vi "NMRvmeCard5.vi"() -> ()   [LabVIEW 2013]
uses:
  <vilib>/Utility/file.llb/Read From Spreadsheet File (DBL).vi
  <vilib>/Analysis/NI_AALBase.lvlib
panel:
  out "Diff Sigma":dbl=0.0014967762883509395 format="%#_13g"
  out "Peak center (MHz)":sgl=213.00838 format="%.3f"
  out "Peak width (MHz)":sgl=0.03243152 format="%.5f"
  in  "Max":bool
  in  "Logoffset (V)":dbl=-5.996000000000003 min=-9.0 max=0.0 step=0.0005 format="%_5g"
  in  "Phase (V)":dbl=6.500000000000002 min=0.0 max=9.0 step=0.0005 format="%_5g"
  out "Telnet error out":errorcluster
  in  "Real/Quad Q curve":bool=TRUE
  out "Temperature (C)":dbl(graph)=27.0
  out "+3V supply":dbl=3.245 format="%_4g"
  out "Temp (C)":dbl=27.0 format="%_4g"
  in  "RemovePed":bool=TRUE
  in  "IF / LOG Det":bool
  in  "Q curve file":string="realback212a.txt"
  out "File name 2":string="C:\\users\\plm\\Desktop\\rssmt\\realback212a.txt"
  in  "AutoTune":bool
  out "RF OK":bool=TRUE
  out "Peak area (V-MHz)":sgl=0.00324335 format="%.5f"
  in  "Gauss Fit":bool
  out "NMR Graph + Fit":cluster{cluster{dbl, "Numeric":dbl}[]}[](graph)=[{[{212.6, "Numeric"=-0.005730750000000197}, {212.60999999999999, "Numeric"=-0.006890750000001482}, {212.62, "Numeric"=-0.003986749999998765}, {212.63, "Numeric"=-0.004218750000000024}, {212.64, "Numeric"=-0.003786750000001219}, {212.65, "Numeric"=-0.004290749999998711}, {212.66, "Numeric"=-0.005430749999999876}, {212.67, "Numeric"=-0.006406750000000973}, {212.68, "Numeric"=-0.005218749999998682}, {212.69, "Numeric"=-0.004966749999999748}, {212.7, "Numeric"=-0.003950750000000758}, {212.71, "Numeric"=-0.0042707499999986775}, {212.72, "Numeric"=-0.004126749999999656}, {212.73, "Numeric"=-0.004318750000000561}, {212.74, "Numeric"=-0.003946750000001408}, {212.75, "Numeric"=-0.00391074999999958}, {212.76, "Numeric"=-0.003910750000000397}, {212.77, "Numeric"=-0.002246750000001148}, {212.78, "Numeric"=-0.002018749999999532}, {212.79, "Numeric"=-0.0012267500000002545}, {212.8, "Numeric"=-0.0017707500000009122}, {212.81, "Numeric"=-0.0019507499999995084}, {212.82, "Numeric"=-0.002066750000000136}, {212.82999999999998, "Numeric"=-0.0013187500000007004}, {212.84, "Numeric"=0.00039325000000048956}, {212.85, "Numeric"=0.00016924999999995416}, {212.85999999999999, "Numeric"=0.0010092499999994845}, {212.87, "Numeric"=1.3250000000461677e-05}, {212.88, "Numeric"=0.0003812500000000196}, {212.89, "Numeric"=0.0014132499999996448}, {212.9, "Numeric"=0.002609250000000409}, {212.91, "Numeric"=0.0036692500000000622}, {212.92, "Numeric"=0.0037932499999997803}, {212.93, "Numeric"=0.0045812500000003325}, {212.94, "Numeric"=0.005733250000000078}, {212.95, "Numeric"=0.007449249999999889}, {212.96, "Numeric"=0.012029250000000227}, {212.97, "Numeric"=0.02267325000000007}, {212.98, "Numeric"=0.03378124999999998}, {212.99, "Numeric"=0.033853249999999946}, {213.0, "Numeric"=0.024589250000000035}, {213.01, "Numeric"=0.021789250000000034}, {213.02, "Numeric"=0.0198532500000001}, {213.03, "Numeric"=0.016981249999999976}, {213.04, "Numeric"=0.01617325000000007}, {213.05, "Numeric"=0.016929250000000225}, {213.06, "Numeric"=0.01484924999999989}, {213.07, "Numeric"=0.015133250000000077}, {213.08, "Numeric"=0.01338125000000033}, {213.09, "Numeric"=0.00949324999999978}, {213.1, "Numeric"=0.007269250000000061}, {213.11, "Numeric"=0.0051092500000004095}, {213.12, "Numeric"=0.004413249999999646}, {213.13, "Numeric"=0.004781250000000021}, {213.14000000000001, "Numeric"=0.0035132500000004613}, {213.15, "Numeric"=0.0027092499999994838}, {213.16, "Numeric"=0.003069249999999955}, {213.17000000000002, "Numeric"=0.004893250000000488}, {213.18, "Numeric"=0.0052812499999992995}, {213.19, "Numeric"=0.0037332499999998625}, {213.2, "Numeric"=0.002549250000000493}, {213.21, "Numeric"=0.003029249999999089}, {213.22, "Numeric"=0.0034732499999997465}, {213.23, "Numeric"=0.0036812500000004663}, {213.24, "Numeric"=0.0035532500000012594}, {213.25, "Numeric"=0.003889249999999604}, {213.26, "Numeric"=0.00258925000000042}, {213.27, "Numeric"=0.0017532500000013032}, {213.28, "Numeric"=0.0021812499999994397}, {213.29, "Numeric"=0.002873250000000347}, {213.3, "Numeric"=0.0024292500000013236}, {213.31, "Numeric"=0.0036492499999992442}, {213.32, "Numeric"=0.003733250000000251}, {213.33, "Numeric"=0.003981250000001318}, {213.34, "Numeric"=0.004593249999999026}, {213.35, "Numeric"=0.0042692500000001245}, {213.36, "Numeric"=0.004509250000001291}, {213.37, "Numeric"=0.004313249999998781}, {213.38, "Numeric"=0.005381249999999974}, {213.39000000000001, "Numeric"=0.006313250000001235}, {213.4, "Numeric"=0.005309249999998517}]}]
  in  "Amp of Q curve":dbl=1.8000000000000034 min=0.0 max=29.0 step=0.01 format="%_3f"
  in  "Subtract Q curve":bool=TRUE
  out "Pedestal Offset":dbl(graph)=0.005806249999999974
  out "Pedestal Difference":dbl(graph)=0.007663500000000241
  out "# Good Spectra":i32=50
  in  "Quality cuts":bool=TRUE
  out "Pedestal OK":bool=TRUE
  out "Sweep #":i32=22
  out "1st Sweep":bool
  out "ADC volts OK":bool=TRUE
  out "Peak Height Distribution":cluster{"Y":dbl[], "Y":dbl[]}[](graph)=[{"Y"=[0.02977452083333331, 0.029831895833333313, 0.02988927083333331, 0.029946645833333313, 0.03000402083333331, 0.030061395833333313, 0.03011877083333331, 0.03017614583333331, 0.030233520833333312, 0.03029089583333331, 0.030348270833333312, 0.03040564583333331, 0.030463020833333312, 0.03052039583333331, 0.030577770833333313, 0.03063514583333331, 0.030692520833333313, 0.03074989583333331, 0.030807270833333313, 0.03086464583333331, 0.03092202083333331, 0.030979395833333312, 0.03103677083333331, 0.031094145833333312, 0.03115152083333331, 0.031208895833333312, 0.03126627083333331, 0.03132364583333331, 0.031381020833333315, 0.03143839583333331, 0.03149577083333331, 0.03155314583333331, 0.03161052083333331, 0.031667895833333314, 0.03172527083333331, 0.03178264583333331, 0.03184002083333331, 0.031897395833333314, 0.03195477083333331, 0.03201214583333331, 0.03206952083333331, 0.032126895833333315, 0.03218427083333331, 0.03224164583333331, 0.03229902083333331, 0.03235639583333331, 0.032413770833333314, 0.03247114583333331, 0.03252852083333331, 0.03258589583333331, 0.032643270833333314, 0.03270064583333331, 0.03275802083333331, 0.03281539583333331, 0.032872770833333315, 0.03293014583333331, 0.03298752083333331, 0.03304489583333331, 0.03310227083333331, 0.033159645833333314, 0.03321702083333331, 0.03327439583333331, 0.03333177083333331, 0.033389145833333314, 0.03344652083333331, 0.03350389583333331, 0.03356127083333331, 0.033618645833333315, 0.03367602083333331, 0.03373339583333331, 0.03379077083333331, 0.03384814583333331, 0.033905520833333314, 0.03396289583333331, 0.03402027083333331, 0.03407764583333331, 0.034135020833333314, 0.03419239583333331, 0.03424977083333331, 0.03430714583333331, 0.034364520833333315, 0.03442189583333331, 0.03447927083333331, 0.03453664583333331, 0.03459402083333331, 0.034651395833333314, 0.03470877083333331, 0.03476614583333331, 0.03482352083333331, 0.034880895833333314, 0.03493827083333331, 0.03499564583333331, 0.03505302083333331, 0.035110395833333315, 0.03516777083333331, 0.03522514583333331, 0.03528252083333331, 0.03533989583333331, 0.035397270833333314, 0.03545464583333331], "Y"=[1.0, 0.0, 0.0, 0.0, 1.0, 0.0, 1.0, 0.0, 0.0, 0.0, 0.0, 0.0, 0.0, 1.0, 0.0, 0.0, 0.0, 0.0, 0.0, 1.0, 0.0, 1.0, 0.0, 0.0, 0.0, 1.0, 1.0, 1.0, 0.0, 1.0, 0.0, 0.0, 0.0, 1.0, 1.0, 0.0, 1.0, 0.0, 2.0, 2.0, 4.0, 0.0, 2.0, 1.0, 1.0, 3.0, 0.0, 0.0, 1.0, 0.0, 1.0, 0.0, 1.0, 1.0, 1.0, 0.0, 0.0, 1.0, 1.0, 0.0, 1.0, 0.0, 1.0, 1.0, 0.0, 1.0, 1.0, 1.0, 0.0, 0.0, 0.0, 0.0, 0.0, 1.0, 2.0, 0.0, 0.0, 1.0, 1.0, 0.0, 0.0, 1.0, 1.0, 0.0, 0.0, 1.0, 0.0, 0.0, 0.0, 0.0, 0.0, 0.0, 0.0, 0.0, 0.0, 0.0, 0.0, 0.0, 0.0, 1.0]}]
  in  "# of Sweeps":i32=50
  out "S/N":dbl=25.80021937658381 format="%_3g"
  out "Peak mean (V)":dbl=0.03249358666666663 format="%_4g"
  out "Peak Height":dbl(graph)=0.033853249999999946
  in  "Raw Data":bool=TRUE
  in  "Tank RF":bool=TRUE
  in  "IF Atten (dB)":i8=3 min=0 max=31 step=1
  in  "IFoffset (V)":dbl=5.450461000000012 min=-0.0 max=9.0 step=0.001 format="%.4f"
  in  "Tune  (V)":dbl=0.3670000000000009 min=-0.5 max=8.0 step=0.001 format="%.4f"
  in  "Hi / Lo Gain":bool
  out "Voltage Array":sgl[](array[numeric])=[0.0296, 0.027, 0.0285, 0.0269, 0.026, 0.0242, 0.0218, 0.0196, 0.0196, 0.0187, 0.0186, 0.0172, 0.0163, 0.0151, 0.0145, 0.0136, 0.0127, 0.0135, 0.0129, 0.0129, 0.0116, 0.0107, 0.0099, 0.01, 0.0111, 0.0103, 0.0106, 0.0091, 0.009, 0.0096, 0.0104, 0.0111, 0.0109, 0.0114, 0.0123, 0.0138, 0.0182, 0.0287, 0.0397, 0.0397, 0.0304, 0.0276, 0.0257, 0.0229, 0.0222, 0.0231, 0.0212, 0.0217, 0.0202, 0.0166, 0.0147, 0.0129, 0.0126, 0.0134, 0.0126, 0.0123, 0.0132, 0.0156, 0.0166, 0.0157, 0.0152, 0.0164, 0.0176, 0.0186, 0.0193, 0.0205, 0.0201, 0.0202, 0.0216, 0.0233, 0.0239, 0.0262, 0.0274, 0.0288, 0.0306, 0.0315, 0.033, 0.0341, 0.0365, 0.0388, 0.0392] format="%.4f"
  in  "Invert Polarity":bool=TRUE
  out "Pedestal Diff (V)":sgl=0.0076635 format="%.3f"
  out "Peak amp (V)":sgl=0.03385325 format="%.3f"
  in  "Save Data to File":bool
  in  "RF Level (dBm)":dbl min=-10.0 max=10.0 step=0.1 format="%.2f"
  out "SMT error out":errorcluster
  out "Sample RMS (V)":dbl=0.0009444444444444443 format="%.4f"
  in  "# Sample/step":i32=80 min=1 max=5000 step=100
  in  "Step Width (MHz)":dbl=0.01 min=0.0 max=1000.0 step=0.0001 format="%.4f"
  in  "Freq Span (MHz)":dbl=0.8 min=0.0 max=3000.0 step=0.1 format="%.3f"
  in  "Center Freq (MHz)":dbl=213.0 min=0.005 max=6000.0 step=0.1 format="%.3f"
  in  "Sweep Mode":u16(ring)=3 items=["Off", "Single", "Auto", "Step"]
  in  "GPIB Addr (28)":refnum<visa-resource-name>="GPIB0::28::INSTR"
  # "E1039 Prototype NMR Control Panel"
  # "Settings"
  # "D\nA\nC"
  # "R\nF\n\nG\nE\nN \n\n+\n\nI\nF"
  # "A\nD\nC"
  # "I\n/\nO"
  # "D\nA\nT\nA\n\nA \nN\nA\nL\nY\nS\nI\nS"
  # "Results"
  # "A\nv\ne\nr\na\ng\ne"
  # "S\nw\ne\ne\np"
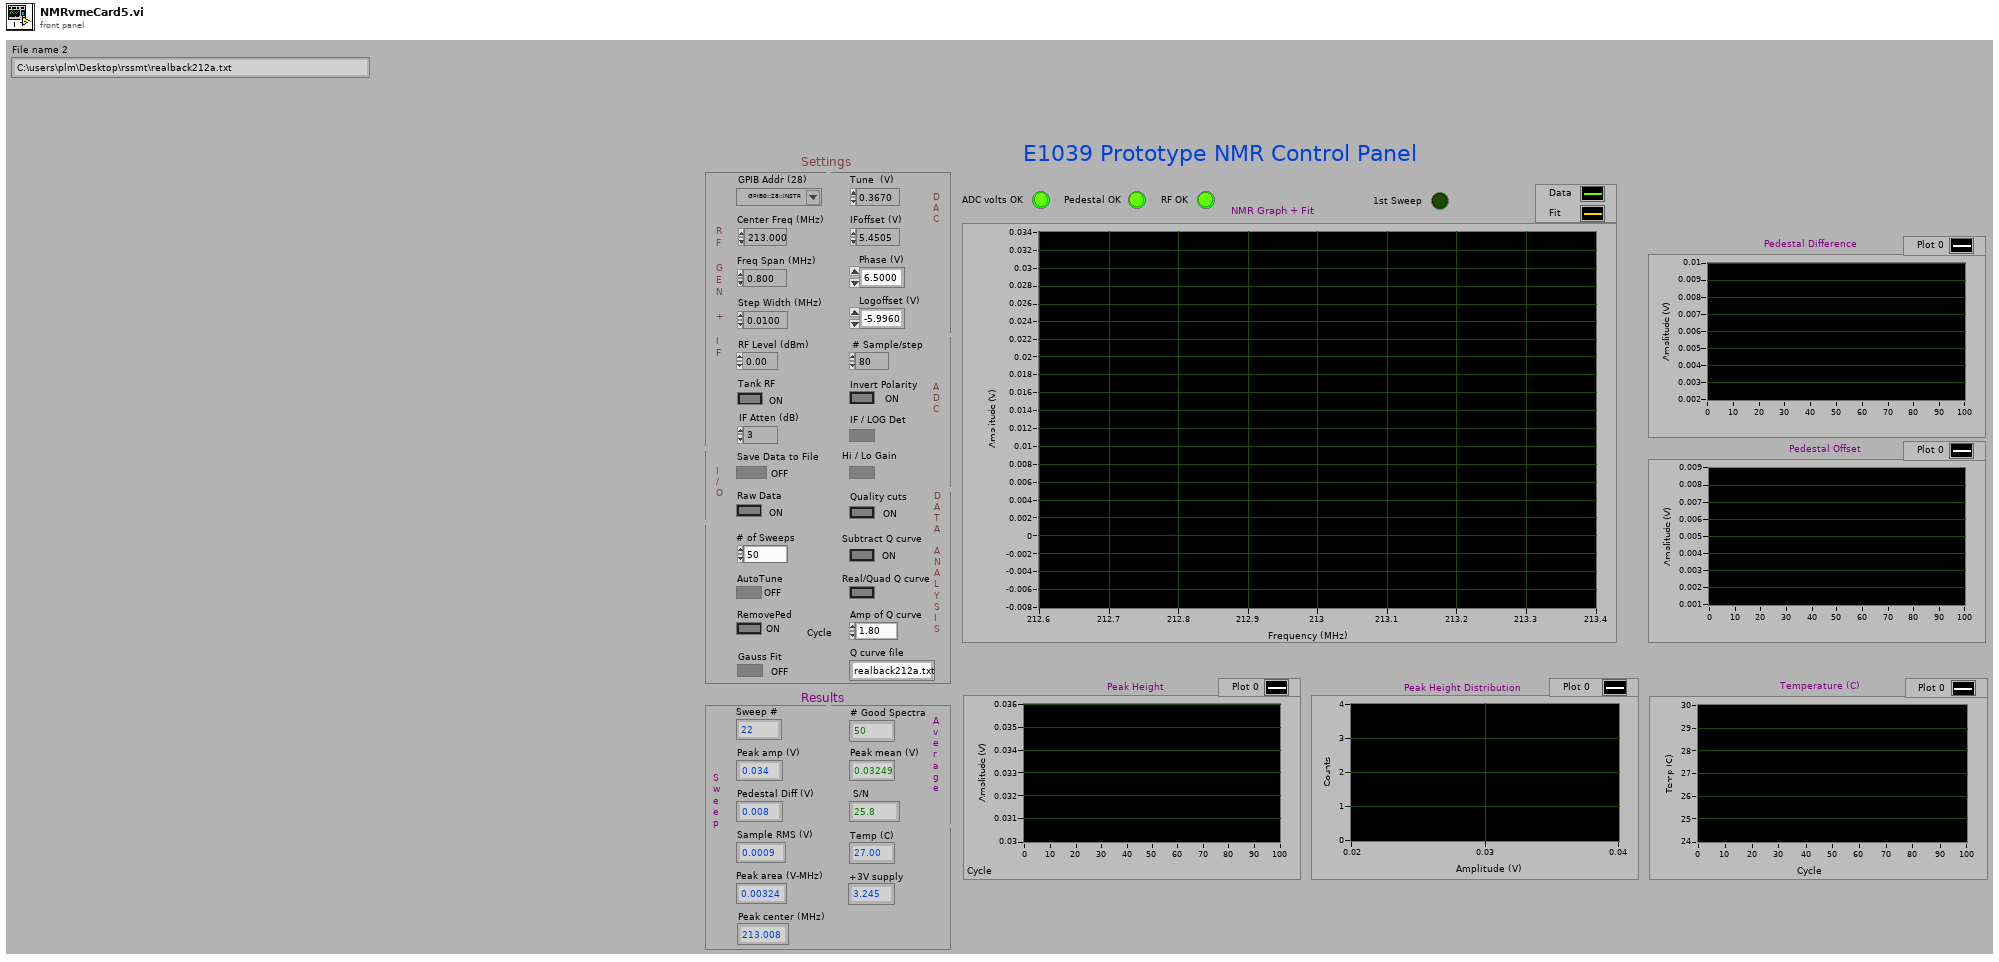
[diagram p1: front panel]
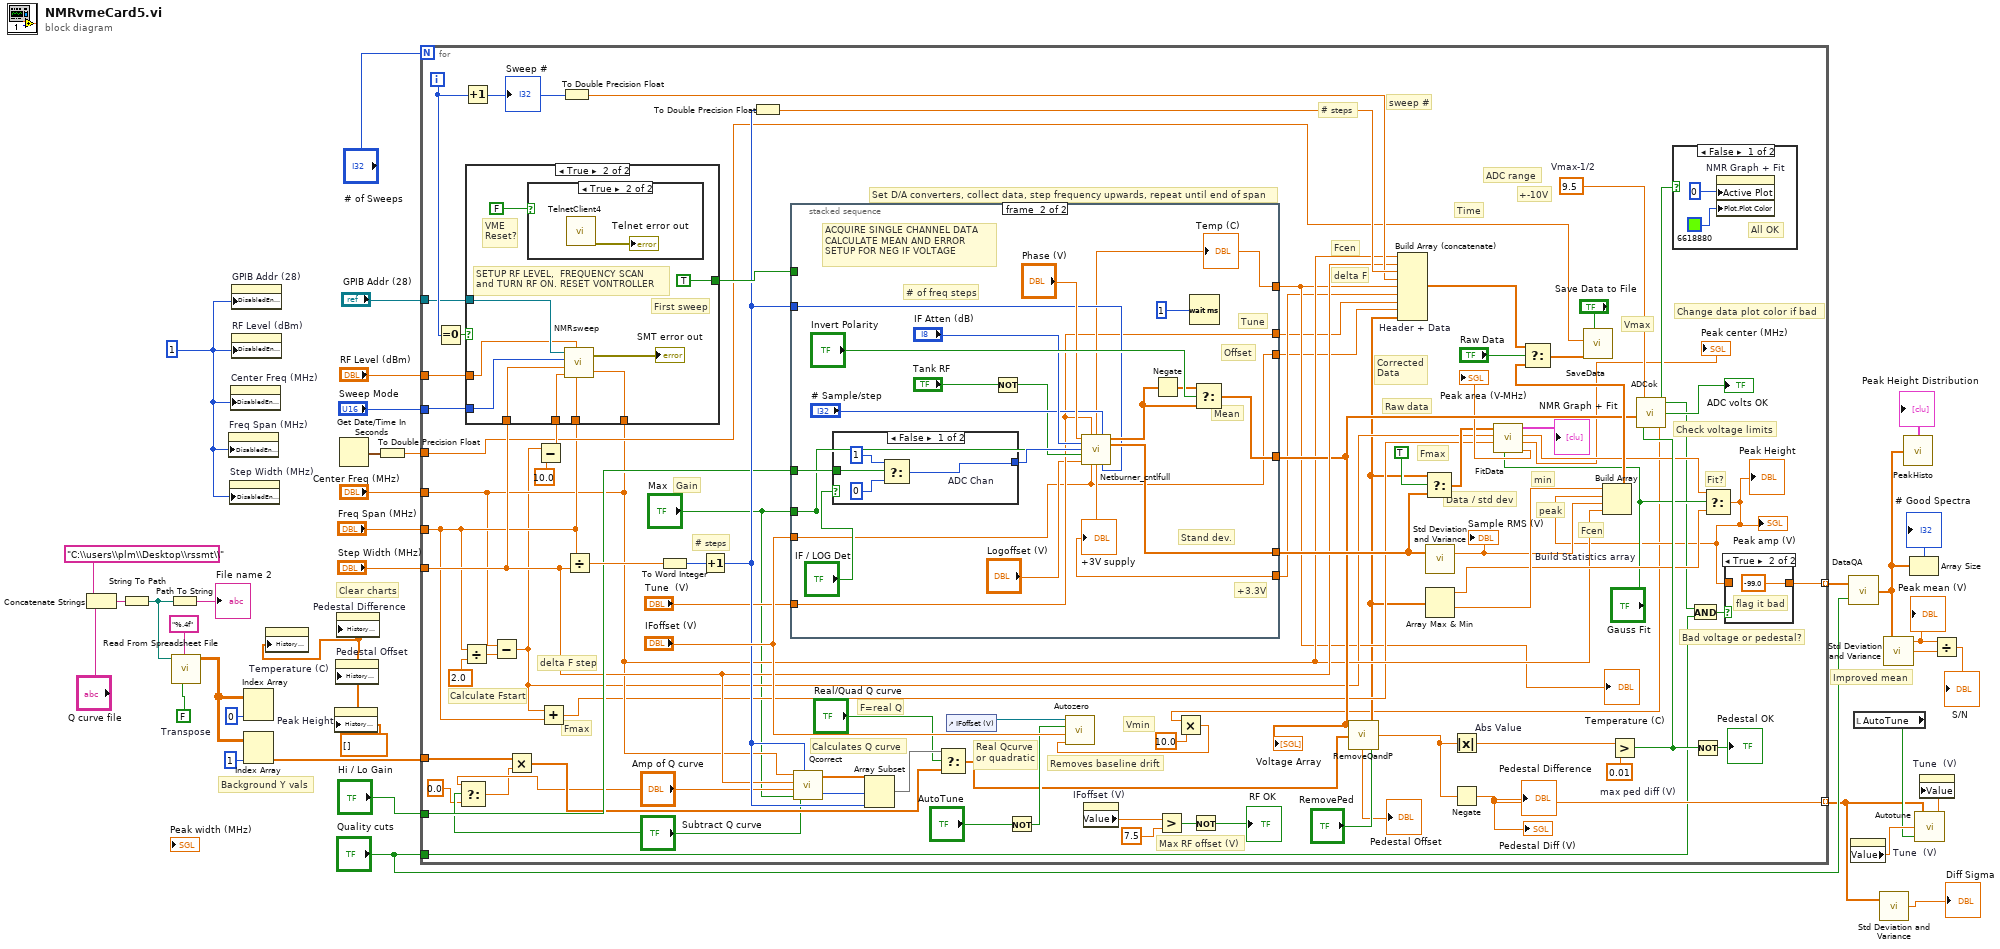
[diagram p0: block diagram]
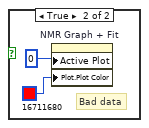
[diagram p2: hidden frame]
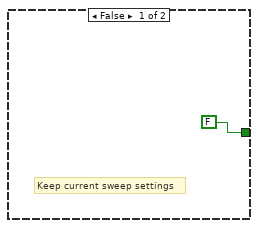
[diagram p4: hidden frame]
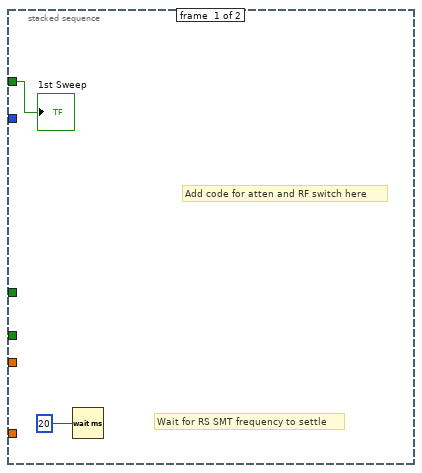
[diagram p6: hidden frame]
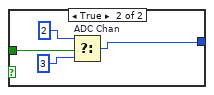
[diagram p7: hidden frame]
diagram:
  w4 = 1
  w16 = FALSE  # Transpose
  w8 = dbl[] []
  # "Background Y vals"
  # "Clear charts"
  # "Improved mean"
  n1 = Concatenate Strings "Concatenate Strings"("C:\\users\\plm\\Desktop\\rssmt\\", "Q curve file") -> (w19:string)
  n2 = String To Path(string=w19) -> (path=w15:path)
  n3 = Path To String(path=w15) -> (string=→"File name 2":string)
  n4 = call-poly <vilib>:"Read From Spreadsheet File.vi"("transpose (no:F)"=w16, "format (%.3f)"="%.4f", "file path (dialog if empty)"=w15) -> ("all rows"=w14:dbl[][])  [unwired: 4 in, 4 out]
  n5 = property on="Freq Span (MHz)" class="DigNum (strict)"("DisabledEnum"=w4) -> ()  [unwired: 2 in, 2 out]
  n6 = property on="Step Width (MHz)" class="DigNum (strict)"("DisabledEnum"=w4) -> ()  [unwired: 2 in, 2 out]
  n7 = property on="Center Freq (MHz)" class="DigNum (strict)"("DisabledEnum"=w4) -> ()  [unwired: 2 in, 2 out]
  n8 = property on="GPIB Addr (28)" class="VISAName"("DisabledEnum"=w4) -> ()  [unwired: 2 in, 2 out]
  n9 = property on="RF Level (dBm)" class="DigNum (strict)"("DisabledEnum"=w4) -> ()  [unwired: 2 in, 2 out]
  n10 = Index Array "Index Array"(array=w14, index (col)=0) -> ()  [unwired: 1 in, 1 out]
  n11 = Index Array(array=w14, index (col)=1) -> (element=w9:dbl[])  [unwired: 1 in]
  n12 = property on="Temperature (C)" class="WFChart (strict)"("History Data"=w8) -> ()  [unwired: 2 in, 2 out]
  n13 = property on="Peak Height" class="WFChart (strict)"("History Data"=w8) -> ()  [unwired: 2 in, 2 out]
  n14 = property on="Pedestal Offset" class="WFChart (strict)"("History Data"=w8) -> ()  [unwired: 2 in, 2 out]
  n15 = property on="Pedestal Difference" class="WFChart (strict)"("History Data"=w8) -> ()  [unwired: 2 in, 2 out]
  n16 = Get Date/Time In Seconds() -> (seconds since 1Jan1904=w21:timestamp)
  n17 = To Double Precision Float(number=w21) -> (double precision float=w20:dbl)
  n18 = for {
    N: "# of Sweeps" -> [_]
    tunnel: [w104] -> w34 mode=indexing
    tunnel: "Quality cuts" -> [w83]
    tunnel: [w88] -> w2 mode=indexing
    tunnel: "Center Freq (MHz)" -> [w70]
    tunnel: "Freq Span (MHz)" -> [w76]
    tunnel: "Step Width (MHz)" -> [w82]
    tunnel: "Sweep Mode" -> [w92]
    tunnel: "Hi / Lo Gain" -> [w91]
    tunnel: "GPIB Addr (28)" -> [w90]
    tunnel: "RF Level (dBm)" -> [w89]
    tunnel: w20 -> [w77]
    tunnel: w9 -> [w55]
    i -> [w102]
    w86 = 9.5  # Vmax-1/2
    w105 = 0.01  # max ped diff (V)
    # "Gain"
    # "F=real Q"
    # "Real Qcurve\nor quadratic"
    # "+-10V"
    # "Vmax"
    # "Change data plot color if bad"
    # "Max RF offset (V)"
    # "Fmax"
    # "Fit?"
    # "Fmax"
    # "Time"
    # "Vmin"
    # "min"
    # "peak"
    # "Raw data"
    # "Corrected\nData"
    # "Fcen"
    # "delta F"
    # "# steps"
    # "ADC range"
    # "sweep #"
    # "Fcen"
    # "Set D/A converters, collect data, step frequency upwards, repeat until end of span"
    # "Calculates Q curve"
    # "Removes baseline drift"
    # "Bad voltage or pedestal?"
    # "Check voltage limits"
    # "Data / std dev"
    # "# steps"
    # "Calculate Fstart"
    # "delta F step"
    n19 = Equal To 0?(x=w102) -> (x = 0?=w107:bool)
    n20 = Select(t="Amp of Q curve", s="Subtract Q curve", f=0.0) -> (s? t:f=w50:dbl)
    n21 = Divide(x=w76, y=sgl 2.0) -> (x/y=w118:dbl)
    n22 = Increment(x=w102) -> (x+1=w93:i32)
    "Sweep #" <- w93
    n23 = Subtract(x=w70, y=w118) -> (x-y=w65:dbl)
    n24 = Multiply(x=w55, y=w50) -> (x*y=w54:dbl[])
    n25 = Subtract(x=w65, y=10.0) -> (x-y=w116:dbl)
    n26 = case shown="True" w107 {
      tunnel: w116 -> [_ w137]
      tunnel: w82 -> [_ w135]
      tunnel: w70 -> [_ w134]
      tunnel: w76 -> [_ w136]
      tunnel: [FALSE TRUE] -> w106
      tunnel: w92 -> [_ w131]
      tunnel: w90 -> [_ w130]
      tunnel: w89 -> [_ w129]
      frame False {
        # "Keep current sweep settings"
      }
      frame True {
        # "VME\nReset?"
        # "First sweep"
        # "SETUP RF LEVEL,  FREQUENCY SCAN\nand TURN RF ON. RESET VONTROLLER"
        n27 = case shown="True" FALSE {
          frame False {
          }
          frame True {
            n28 = call "TelnetClient4.vi"() -> ("Telnet error"=→"Telnet error out":errorcluster)  [unwired: 4 in, 3 out]
          }
        }
        n29 = call "NMRsweep.vi"("Center Freq (MHz)"=w134, "Freq Span (MHz)"=w136, "RF Level (dBm)"=w129, "Foffset (MHz)"=w137, "Step Width (MHz)"=w135, "Sweep Mode"=w131, "GPIB Addr (28)"=w130) -> ("error out"=→"SMT error out":errorcluster)
      }
    }
    n30 = Add(x=w65, y=w76) -> (x+y=w64:dbl)
    n31 = To Double Precision Float(number=w93) -> (double precision float=w94:dbl)
    n32 = Divide(x=w76, y=w82) -> (x/y=w120:dbl)
    n33 = To Word Integer(number=w120) -> (16bit integer=w117:i16)
    n34 = Increment(x=w117) -> (x+1=w96:i16)
    n35 = To Double Precision Float(number=w96) -> (double precision float=w95:dbl)
    n36 = stacked-sequence {
      tunnel: [_ w152] -> w110
      tunnel: [_ w159] -> w80
      tunnel: w96 -> [_ w149]
      tunnel: "IFoffset (V)" -> [_ w142]
      tunnel: w91 -> [_ w157]
      tunnel: w106 -> [w139 _]
      tunnel: "Tune  (V)" -> [_ w144]
      tunnel: [_ w148] -> w46
      tunnel: [_ w145] -> w45
      tunnel: [_ w144] -> w43
      tunnel: [_ w142] -> w42
      tunnel: [_ w141] -> _
      tunnel: "Max" -> [_ w141]
      frame #0 {
        # "Add code for atten and RF switch here"
        # "Wait for RS SMT frequency to settle"
        n37 = Wait (ms)(milliseconds to wait=20) -> ()  [unwired: 1 out]
        "1st Sweep" <- w139
      }
      frame #1 {
        # "+3.3V"
        # "Offset"
        # "Tune"
        # "Stand dev."
        # "Mean"
        # "ACQUIRE SINGLE CHANNEL DATA\nCALCULATE MEAN AND ERROR\nSETUP FOR NEG IF VOLTAGE"
        # "# of freq steps"
        n38 = case shown="False" "IF / LOG Det" {
          tunnel: w157 -> [w165 w166]
          tunnel: [w162 w167] -> w151
          frame False {
            n39 = Select "ADC Chan"(t=1, s=w165, f=0) -> (s? t:f=w162:i32)
          }
          frame True {
            n40 = Select "ADC Chan"(t=2, s=w166, f=3) -> (s? t:f=w167:i32)
          }
        }
        n41 = Not(x="Tank RF") -> (.not. x?=w147:bool)
        n42 = call "Netburner_cntlfull.vi"("Phase Volt"="Phase (V)", "Tune Volt"=w144, "# Data"="# Sample/step", "IF Atten (dB)"="IF Atten (dB)", "NMR ADC"=w151, "Hi Gain"=w141, "Tank RF"=w147, "LogOff Volt"="Logoffset (V)", "IFOff Volt"=w142, "# f steps"=w149) -> ("Temp (C)"=w148:dbl, "ADC value"=w153:dbl[], "ADC error"=w152:dbl[], "Volts"=w145:dbl)  [unwired: 2 out]
        "Temp (C)" <- w148
        "+3V supply" <- w145
        n43 = Negate(x=w153) -> (-x=w158:dbl[])
        n44 = Wait (ms)(milliseconds to wait=1) -> ()  [unwired: 1 out]
        n45 = Select(t=w158, s="Invert Polarity", f=w153) -> (s? t:f=w159:dbl[])
      }
    }
    "Voltage Array" <- w80
    "Temperature (C)" <- w46
    n46 = call "Qcorrect.vi"("Subtract Q curve"="Subtract Q curve", "Nstep"=w96, "Max Gain"="Max", "Amp of Q curve"="Amp of Q curve", "Step Width (MHz)"=w82, "Center Freq (MHz)"=w70) -> ("Start"=w111:i32, "Array"=w112:dbl[])
    n47 = Array Subset "Array Subset"(array=w112, index=w111, length=w96) -> (w58:dbl[])
    n48 = Select(t=w58, s="Real/Quad Q curve", f=w54) -> (s? t:f=w57:dbl[])
    n49 = control-ref of="IFoffset (V)"() -> (w85:refnum<vi>)
    n50 = Not(x="AutoTune") -> (.not. x?=w59:bool)
    n51 = property on="IFoffset (V)" class="DigNum (strict)"() -> ("Value"=w74:dbl)  [unwired: 2 in, 2 out]
    n52 = Greater?(x=w74, y=7.5) -> (0:w72:bool)
    n53 = Not(x=w72) -> (.not. x?=→"RF OK":bool)
    n54 = call "RemoveQandP.vi"("Subtract Ped?"="RemovePed", "Qcurve"=w57, "Raw data"=w80) -> ("Ped L-R"=w98:dbl, "Corrected data"=w44:dbl[], "Ped Offfset"=→"Pedestal Offset":dbl)
    n55 = Build Array (concatenate) "Header + Data"(w70, w82, w95, w94, w46, w45, w43, w42, w44) -> (w97:dbl[])
    n56 = Select(t=w44, s=TRUE, f=w110) -> (s? t:f=w66:dbl[])
    n57 = call <vilib>:"Std Deviation and Variance.vi"("X"=w110) -> ("mean"=w81:dbl)  [unwired: 1 in, 2 out]
    "Sample RMS (V)" <- w81
    n58 = Array Max & Min(array=w44) -> (max value=w75:dbl, min value=w109:dbl)  [unwired: 2 out]
    n59 = Absolute Value "Abs Value"(x=w98) -> (abs(x)=w100:dbl)
    n60 = Negate(x=w98) -> (-x=w88:dbl)
    "Pedestal Diff (V)" <- w88
    "Pedestal Difference" <- w88
    n61 = call "FitData.vi"("Fit?"="Gauss Fit", "Fmax"=w64, "Fmin"=w65, "Yarray"=w66) -> ("Peak Area (V-MHz)"=→"Peak area (V-MHz)":dbl, "Center Freq (MHz)"=→"Peak center (MHz)":dbl, "Amplitude (V)"=w68:dbl, "NMR Graph + Fit"=→"NMR Graph + Fit":cluster{cluster{dbl, "Numeric":dbl}[]}[])  [unwired: 1 out]
    n62 = Greater?(x=w100, y=w105) -> (0:w87:bool)
    n63 = call "ADCok.vi"("PedOK"=w87, "Array"=w80, "Vmax-1/2"=w86) -> ("Vmin"=w39:dbl, "ADC voltages OK"=→"ADC volts OK":bool, "Allok"=w62:bool)
    n64 = Multiply(x=w39, y=10.0) -> (x*y=w37:dbl)
    n65 = call "Autozero.vi"("Vmin (V)"=w37, "IFoffset (V)"="IFoffset (V)", "Enable"=w59, "reference"=w85) -> ()
    n66 = case shown="False" w62 {
      frame False {
        # "All OK"
        n67 = property on="NMR Graph + Fit" class="XYGraph (strict)"("Active Plot"=0, "Plot.Plot Color"=u32 6618880) -> ()  [unwired: 2 in, 2 out]
      }
      frame True {
        # "Bad data"
        n68 = property on="NMR Graph + Fit" class="XYGraph (strict)"("Active Plot"=0, "Plot.Plot Color"=u32 16711680) -> ()  [unwired: 2 in, 2 out]
      }
    }
    n69 = And(x=w62, y=w83) -> (x .and. y?=w101:bool)
    n70 = Not(x=w87) -> (.not. x?=→"Pedestal OK":bool)
    n71 = Select(t=w68, s="Gauss Fit", f=w75) -> (s? t:f=w61:dbl)
    "Peak amp (V)" <- w61
    "Peak Height" <- w61
    n72 = Build Array "Build Statistics array"(w109, w61, w81, w70) -> (w115:dbl[])
    n73 = Select(t=w97, s="Raw Data", f=w115) -> (s? t:f=w78:dbl[])
    n74 = call "SaveData.vi"("Array"=w78, "Save Data to File"="Save Data to File", "Ext time (sec)"=w77) -> ()  [unwired: 1 out]
    n75 = case shown="True" w101 {
      tunnel: [w125 -99.0] -> w104
      tunnel: w61 -> [w125 _]
      frame False {
        # "Data OK"
      }
      frame True {
        # "flag it bad"
      }
    }
  }
  n76 = call "DataQA.vi"("Quality cuts"="Quality cuts", "Data In"=w34) -> ("Data Out"=w33:dbl[])
  n77 = property on="Tune  (V)" class="DigNum (strict)"() -> ("Value"=w24:dbl)  [unwired: 2 in, 2 out]
  n78 = local read "AutoTune"() -> (w3:bool)
  n79 = call <vilib>:"Std Deviation and Variance.vi"("X"=w2) -> ("standard deviation"=→"Diff Sigma":dbl)  [unwired: 1 in, 2 out]
  n80 = call <vilib>:"Std Deviation and Variance.vi"("X"=w33) -> ("mean"=w7:dbl, "standard deviation"=w6:dbl)  [unwired: 1 in, 1 out]
  "Peak mean (V)" <- w7
  n81 = call "PeakHisto.vi"("Data Out"=w33) -> ("XY Graph"=→"Peak Height Distribution":cluster{"Y":dbl[], "Y":dbl[]}[])
  n82 = Array Size(array=w33) -> (size(s)=→"# Good Spectra":i32)
  n83 = call "Autotune.vi"("Adjust Tune"=w3, "Tune Vin"=w24, "Pedestal Diff"=w2) -> ("Tune Vout"=w23:dbl)
  n84 = property on="Tune  (V)" class="DigNum (strict)"("Value"=w23) -> ()  [unwired: 2 in, 2 out]
  n85 = Divide(x=w7, y=w6) -> (x/y=→"S/N":dbl)
